vi "dialog test.vi"() -> ()   [LabVIEW 2010]
panel:
  out "data":bool
  out "in counting loop":bool
  out "counter":i32
  in  "stop":bool
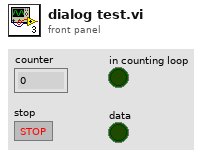
[diagram p1: front panel]
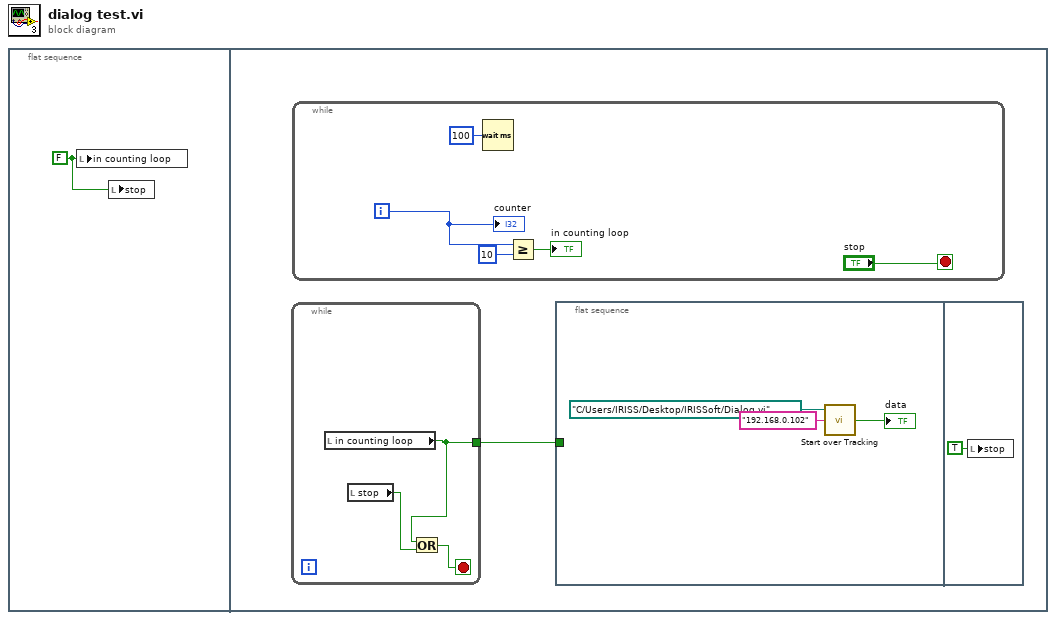
[diagram p0: block diagram]
diagram:
  n1 = flat-sequence {
    frame #0 {
      w1 = FALSE ("in counting loop")
      n2 = local write "in counting loop"(w1) -> ()
      n3 = local write "stop"(w1) -> ()
    }
    frame #1 {
      n4 = while {
        tunnel: [w7] -> w2
        stop <- w9 stop-if-true
        n5 = local read "in counting loop"() -> (w7:bool)
        n6 = local read "stop"() -> (w8:bool)
        n7 = Or(x=w7, y=w8) -> (x .or. y?=w9:bool)
      }
      n8 = while {
        i -> [w10]
        stop <- "stop" stop-if-true
        n9 = Wait (ms)(milliseconds to wait=u32 100) -> ()  [unwired: 1 out]
        n10 = Greater Or Equal?(x=w10, y=10) -> (x >= y?=→"in counting loop":bool)
        "counter" <- w10
      }
      n11 = flat-sequence {
        tunnel: w2 -> [_]
        frame #0 {
          n12 = call "Start over Tracking.vi"("Host System IP Address"="192.168.0.102", "VI Path on Host"=path "C:/Users/IRISS/Desktop/IRISSoft/Dialog.vi" ("vi path")) -> ("yes/no?"=→"data":bool)  [unwired: 2 in, 1 out]
        }
        frame #1 {
          n13 = local write "stop"(TRUE ("stop")) -> ()
        }
      }
    }
  }
